vi "set_remote-interface-mode.vi"(8 "error in (no error)":errorcluster, 10 "mode":u16(ring) items=["local", "remote", "remot with lock-out"], 11 "Agilent 34980A in":refnum<class "Agilent 34980A.lvclass">) -> (0 "error out":errorcluster, 3 "Agilent 34980A out":refnum<class "Agilent 34980A.lvclass">)   [LabVIEW 2017, in "Agilent 34980A.lvclass"]
doc: "sets the remote interface of the actual instrument.\nMode=1 (local), 2 (remote), 3 (remote with lockout)"
uses:
  Agilent 34980A.lvclass
  instrument.lvclass
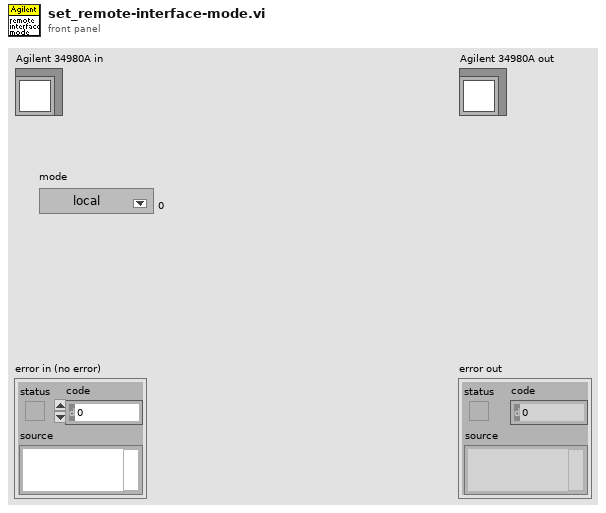
[diagram p1: front panel]
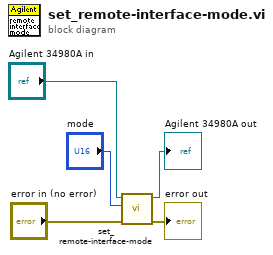
[diagram p0: block diagram]
diagram:
  n1 = call-parent "set_remote-interface-mode.vi"("error in (no error)"="error in (no error)", "mode"="mode", "instrument in"="Agilent 34980A in") -> ("error out"=→"error out":errorcluster, "instrument out"=→"Agilent 34980A out":refnum<class "Agilent 34980A.lvclass">)  [unwired: 7 in]
